vi "Retira_tudo_depois_da_virgula.vi"(1 "Entrada":string) -> (0 "Saída":string)   [LabVIEW 2018]
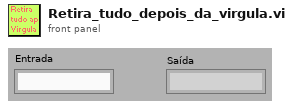
[diagram p1: front panel]
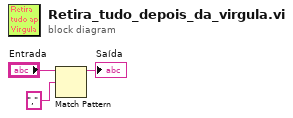
[diagram p0: block diagram]
diagram:
  n1 = Match Pattern(string="Entrada", regular expression=",") -> (before substring=→"Saída":string)  [unwired: 1 in, 3 out]
